vi "Read T controller configuration.vi"(8 "error in (no error)":errorcluster, 11 "Temperature Controller Driver in":refnum<class "Temperature Controller Driver.lvclass">) -> (0 "error out":errorcluster, 2 "Configuration":T1={"Record Channels"=["A"], "Add raw signal"=FALSE, "New set point"=0.0, "Record heater"=FALSE}, 3 "Temperature Controller Driver out":refnum<class "Temperature Controller Driver.lvclass">)   [LabVIEW 2019, in "Temperature Controller Driver.lvclass"]
uses:
  Temperature Controller Driver.lvclass
  C:/GitHub/NHMFL_Core/Libraries/Instruments/Instrument Driver/Instrument Driver.lvclass
  T controller configuration.ctl
  Instrument Driver/Read User configuration.vi
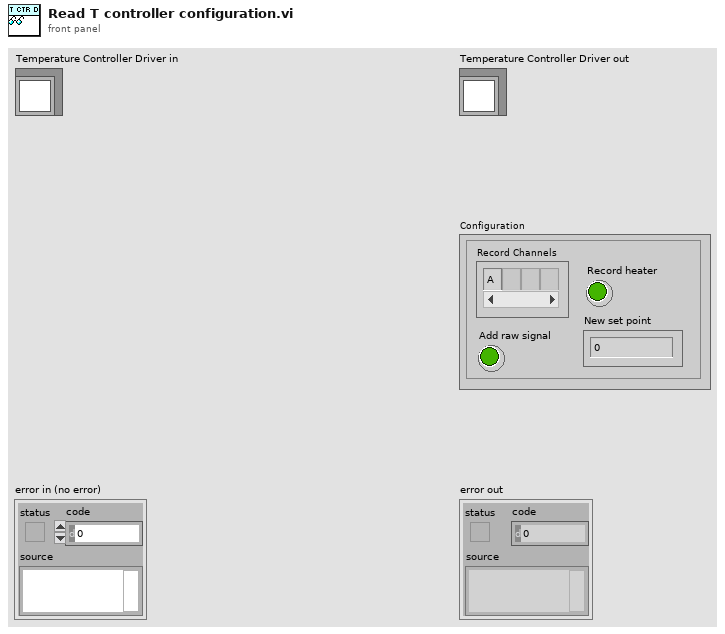
[diagram p1: front panel]
types:
  T1 = typedef "T controller configuration.ctl" = cluster{"Record Channels":string[], "Add raw signal":bool, "New set point":dbl, "Record heater":bool}
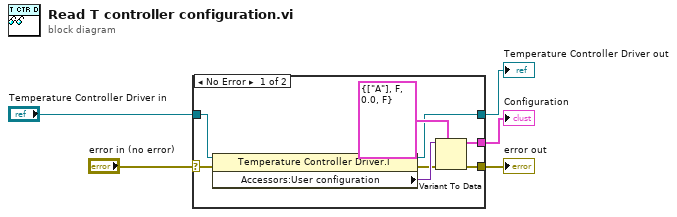
[diagram p0: block diagram]
diagram:
  n1 = case shown="No Error" "error in (no error)" {
    selector: "error in (no error)" -> [w7 w14]
    tunnel: [w6 w14] -> w4
    tunnel: [w10 w15] -> w2
    tunnel: "Temperature Controller Driver in" -> [w13 w15]
    tunnel: [w11 _] -> w1
    frame No Error {
      n2 = property class="Temperature Controller Driver.l"(reference=w13, error in=w7) -> (reference out=w10:refnum<class "Temperature Controller Driver.lvclass">, error out=w8:errorcluster, "Accessors:User configuration"=w9:variant)
      n3 = Variant To Data(error in=w8, type=T1 {"Record Channels"=["A"], "Add raw signal"=FALSE, "New set point"=0.0, "Record heater"=FALSE} ("Configuration"), Variant=w9) -> (data=w11:T1, error out=w6:errorcluster)
    }
    frame Error {
    }
  }
  "error out" <- w4
  "Temperature Controller Driver out" <- w2
  "Configuration" <- w1
